vi "Rem_Raw_DF.vi"(1 "Clear History?":bool, 2 "Filename to Remember":path) -> (0 "List of Filenames":path[](array[path]))   [LabVIEW 2010]
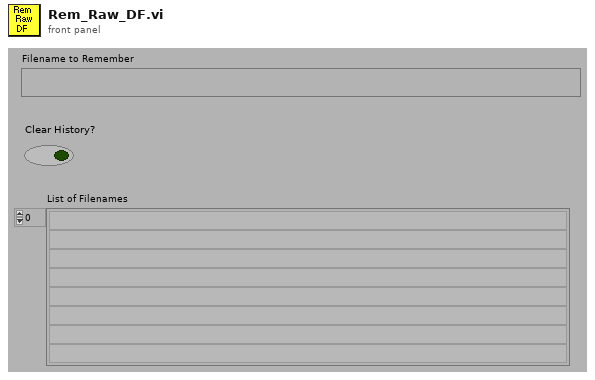
[diagram p1: front panel]
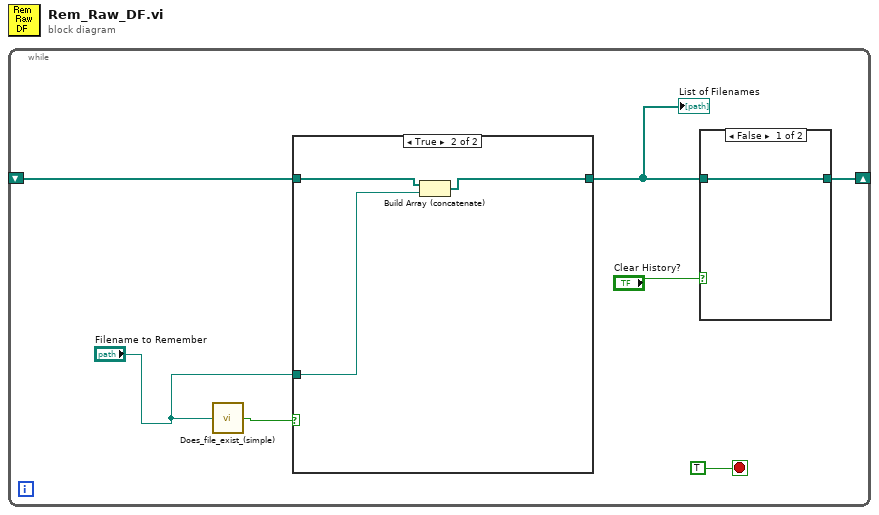
[diagram p0: block diagram]
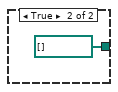
[diagram p2: hidden frame]
diagram:
  n1 = while {
    shift-right: [w2] -> _
    shift-left: _ -> [w7]
    stop <- TRUE stop-if-true
    n2 = call "Does_file_exist_(simple).vi"("Pathname"="Filename to Remember") -> ("exists?"=w4:bool)
    n3 = case shown="True" w4 {
      tunnel: w7 -> [w10 w13]
      tunnel: "Filename to Remember" -> [_ w12]
      tunnel: [w10 w11] -> w1
      frame False {
      }
      frame True {
        n4 = Build Array (concatenate)(w13, w12) -> (w11:path[])
      }
    }
    "List of Filenames" <- w1
    n5 = case shown="False" "Clear History?" {
      tunnel: w1 -> [w8 _]
      tunnel: [w8 path[] []] -> w2
      frame False {
      }
      frame True {
      }
    }
  }
